vi "Read Actual Server Identity.vi"(10 "server errors":string, 11 "client in":refnum<class "Generic Client.lvclass">) -> (2 "fingerprint":string, 3 "client out":refnum<class "Generic Client.lvclass">)   [LabVIEW 2020, in "NI_SSH.lvlib" / "Generic Client.lvclass"]
uses:
  <vilib>/net/SSH/Client/Generic/Generic Client.lvclass
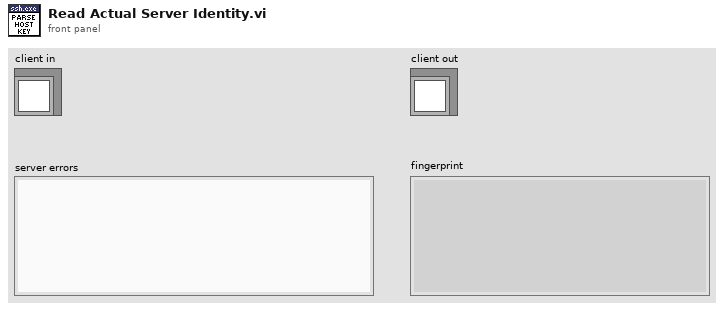
[diagram p1: front panel]
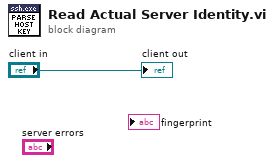
[diagram p0: block diagram]
diagram:
  "client out" <- "client in"
